vi "Climb_Test.vi"(11 "Joystick_In":T1) -> ()   [LabVIEW 2019]
uses:
  Subsystems/Climb/Climb_Pivot/Climb_Pivot_Control_States.ctl
  Subsystems/Climb/Climb_Pivot/Climb_Pivot_Cluster.ctl
  Subsystems/Climb/Climb_Transverse/Climb_Transverse_Control_States.ctl
  Subsystems/Climb/Climb_Transverse/Climb_Transverse_Cluster.ctl
  Subsystems/Climb/Climb_Elevator/Climb_Elevator_Control_States.ctl
  Subsystems/Climb/Climb_Elevator/Climb_Elevator_Cluster.ctl
  Globals/Climb_Globals.vi
  Utility_VIs/Joystick_Controls.ctl
panel:
  in  "Pivot_Speed":dbl=1.0
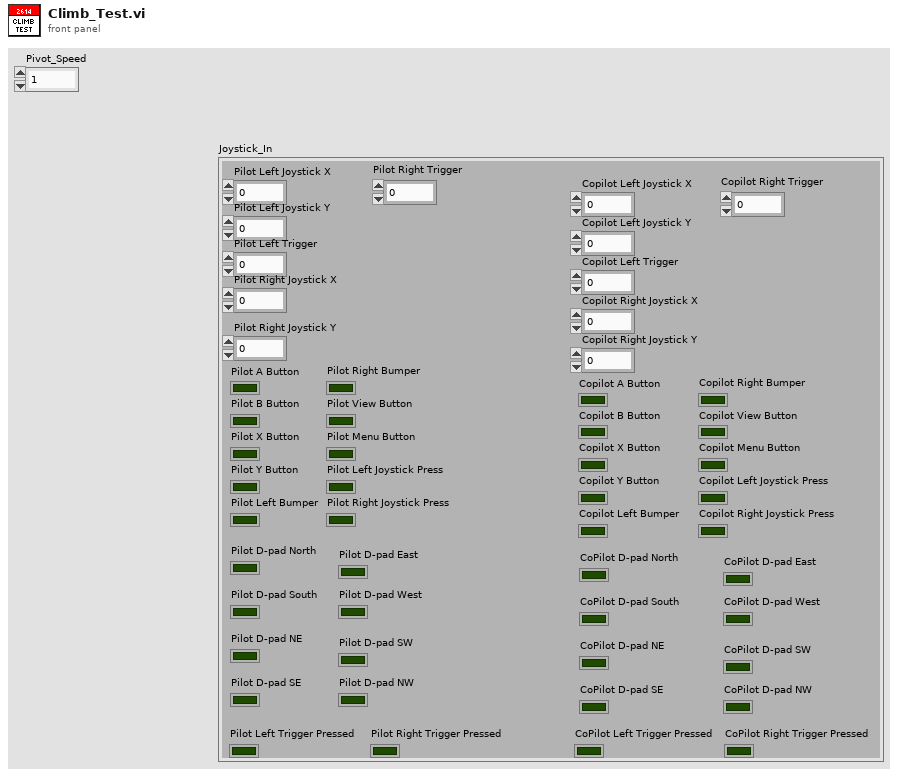
[diagram p1: front panel]
types:
  T1 = typedef "Joystick_Controls.ctl" = cluster{"Pilot Left Joystick X":dbl, "Pilot Left Joystick Y":dbl, "Pilot A Button":bool, "Pilot B Button":bool, "Pilot X Button":bool, "Pilot Y Button":bool, "Pilot Left Bumper":bool, "Pilot Right Bumper":bool, "Pilot View Button":bool, "Pilot Menu Button":bool, "Pilot Left Joystick Press":bool, "Pilot Right Joystick Press":bool, "Pilot Left Trigger":dbl, "Pilot Right Joystick X":dbl, "Pilot Right Joystick Y":dbl, "Pilot Right Trigger":dbl, "Copilot Left Joystick X":dbl, "Copilot Left Joystick Y":dbl, "Copilot A Button":bool, "Copilot B Button":bool, "Copilot X Button":bool, "Copilot Y Button":bool, "Copilot Left Bumper":bool, "Copilot Right Bumper":bool, "Copilot View Button":bool, "Copilot Menu Button":bool, "Copilot Left Joystick Press":bool, "Copilot Right Joystick Press":bool, "Copilot Left Trigger":dbl, "Copilot Right Joystick X":dbl, "Copilot Right Joystick Y":dbl, "Copilot Right Trigger":dbl, "Pilot D-pad North":bool, "Pilot D-pad South":bool, "Pilot D-pad East":bool, "Pilot D-pad West":bool, "Pilot D-pad NE ":bool, "Pilot D-pad SE":bool, "Pilot D-pad SW":bool, "Pilot D-pad NW":bool, "CoPilot D-pad North":bool, "CoPilot D-pad South":bool, "CoPilot D-pad East":bool, "CoPilot D-pad West":bool, "CoPilot D-pad NE":bool, "CoPilot D-pad SE":bool, "CoPilot D-pad SW":bool, "CoPilot D-pad NW":bool, "Pilot Left Trigger Pressed":bool, "Pilot Right Trigger Pressed":bool, "CoPilot Left Trigger Pressed":bool, "CoPilot Right Trigger Pressed":bool}
  T2 = typedef "Climb_Elevator_Cluster.ctl" = cluster{"Extend?":bool, "Elevator_Throttle":dbl, "Control_States":T3}
  T3 = typedef "Climb_Elevator_Control_States.ctl" = enum16{"No-Op", "Brake", "Going_Up", "Going_Down", "Manual"}
  T4 = typedef "Climb_Transverse_Cluster.ctl" = cluster{"Auto-Balance?":bool, "Transverse_Throttle":dbl, "Control_States":T5}
  T5 = typedef "Climb_Transverse_Control_States.ctl" = enum16{"No-Op", "Manual", "Auto-Balancing"}
  T6 = typedef "Climb_Pivot_Cluster.ctl" = cluster{"Up?":bool, "Pivot_Throttle":dbl, "Control_States":T7}
  T7 = typedef "Climb_Pivot_Control_States.ctl" = enum16{"No-Op", "Moving_Down", "Moving_Up", "Manual"}
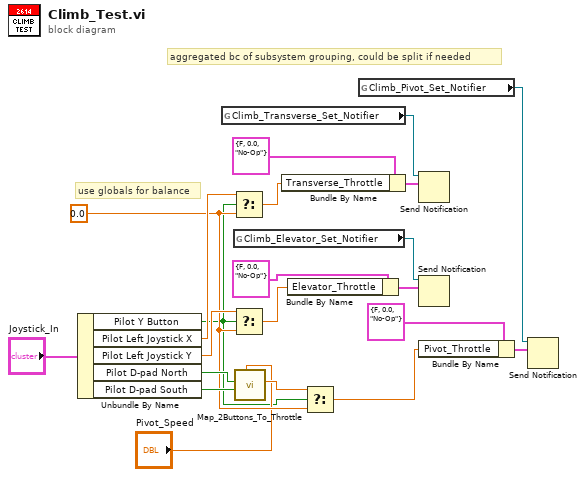
[diagram p0: block diagram]
diagram:
  w15 = 0.0 ("f")
  # "aggregated bc of subsystem grouping, could be split if needed"
  # "use globals for balance"
  n1 = Unbundle By Name("Joystick_In") -> ("Pilot Y Button"=w1:bool, "Pilot Left Joystick X"=w20:dbl, "Pilot Left Joystick Y"=w19:dbl, "Pilot D-pad North"=w18:bool, "Pilot D-pad South"=w17:bool)
  n2 = global read "Climb_Globals.vi" "Climb_Transverse_Set_Notifier"() -> (w7:refnum<notifier>)
  n3 = Select(t=w20, s=w1, f=w15) -> (s? t:f=w8:dbl)
  n4 = global read "Climb_Globals.vi" "Climb_Elevator_Set_Notifier"() -> (w6:refnum<notifier>)
  n5 = Select(t=w19, s=w1, f=w15) -> (s? t:f=w9:dbl)
  n6 = call "Map_2Buttons_To_Throttle.vi"("Power"="Pivot_Speed", "Down"=w17, "Up"=w18) -> ("Throttle"=w16:dbl)  [unwired: 8 in]
  n7 = Bundle By Name(cluster=T4 {"Auto-Balance?"=FALSE, "Transverse_Throttle"=0.0, "Control_States"=enum."No-Op"} ("Climb_Transverse_Cluster"), "Transverse_Throttle"=w8) -> (w2:T4)
  n8 = Bundle By Name(cluster=T2 {"Extend?"=FALSE, "Elevator_Throttle"=0.0, "Control_States"=enum."No-Op"} ("Climb_Pivot_Cluster"), "Elevator_Throttle"=w9) -> (w3:T2)
  n9 = Select(t=w16, s=w1, f=w15) -> (s? t:f=w10:dbl)
  n10 = global read "Climb_Globals.vi" "Climb_Pivot_Set_Notifier"() -> (w5:refnum<notifier>)
  n11 = Send Notification(notification=w2, notifier=w7) -> ()  [unwired: 1 in, 2 out]
  n12 = Send Notification(notification=w3, notifier=w6) -> ()  [unwired: 1 in, 2 out]
  n13 = Bundle By Name(cluster=T6 {"Up?"=FALSE, "Pivot_Throttle"=0.0, "Control_States"=enum."No-Op"} ("Climb_Pivot_Cluster"), "Pivot_Throttle"=w10) -> (w4:T6)
  n14 = Send Notification(notification=w4, notifier=w5) -> ()  [unwired: 1 in, 2 out]
